vi "CalcArea.vi"(8 "Error In":errorcluster, 11 "Square in":refnum<class "Square.lvclass">) -> (0 "Error Out":errorcluster, 2 "Area":dbl, 3 "Square out":refnum<class "Square.lvclass">)   [LabVIEW 2021, in "Square.lvclass"]
doc: "Calc a area of square object."
uses:
  Square.lvclass
  Rectangle/Rectangle.lvclass
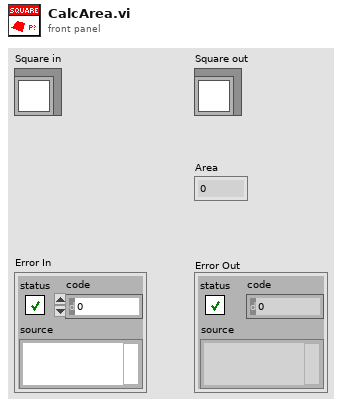
[diagram p1: front panel]
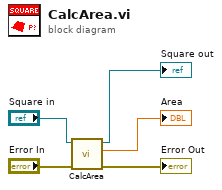
[diagram p0: block diagram]
diagram:
  n1 = call-parent "CalcArea.vi"("Error In"="Error In", "Rectangle in"="Square in") -> ("Error Out"=→"Error Out":errorcluster, "Area"=→"Area":dbl, "Rectangle out"=→"Square out":refnum<class "Square.lvclass">)  [unwired: 7 in]
